vi "Set First Timestamp.vi"(8 "error in (no error)":errorcluster, 11 "Waveform Generator in":refnum<class "Waveform Generator.lvclass">) -> (0 "error out":errorcluster, 3 "Waveform Generator out":refnum<class "Waveform Generator.lvclass">)   [LabVIEW 2015, in "Waveform Generator.lvclass"]
uses:
  Waveform Generator.lvclass
  Waveform Generator.lvclass/Waveform Generator.ctl
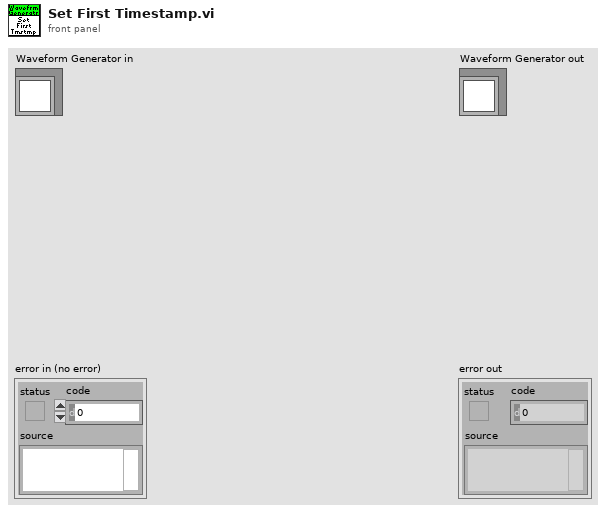
[diagram p1: front panel]
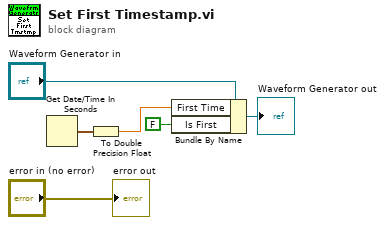
[diagram p0: block diagram]
diagram:
  n1 = Get Date/Time In Seconds() -> (seconds since 1Jan1904=w3:timestamp)
  n2 = To Double Precision Float(number=w3) -> (double precision float=w2:dbl)
  n3 = Bundle By Name(cluster="Waveform Generator in", "First Time"=w2, "Is First"=FALSE ("IsFirst")) -> (→"Waveform Generator out":refnum<class "Waveform Generator.lvclass">)
  "error out" <- "error in (no error)"
